vi "Maintenance v0.3.vi"(8 "Error In":errorcluster) -> (0 "Error out":errorcluster)   [LabVIEW 2017]
uses:
  GV/Maintenance GV.vi
panel:
  out "ICS_BF_Low_Level_1":bool
  in  "SOL_Index_CNVR_Output _Separator _Rear":bool
  out "RS_Measurement_2_Rear":bool
  out "RS_Measurement_3_Rear":bool
  out "RS_Measurement_4_Rear":bool
  out "RS_Measure_Clamp_Rear":bool
  in  "DO1.19":bool
  in  "Continuous?":bool
  out "DI2.25":bool
  out "DI2.26":bool
  out "DI2.31":bool
  out "DI2.30":bool
  out "DI2.29":bool
  out "DI2.28":bool
  out "DI2.27":bool
  in  "Main Tab":T1(tab)
  out "SW_Door_Front":bool
  in  "DO1.31":bool
  in  "DO1.30":bool
  out "Machine_ON":bool
  out "E_stop":bool
  out "SW_Pressure":bool
  out "SW_Start":bool
  out "SW_Reset":bool
  out "SW_Stop":bool
  out "SW_Door_Rear":bool
  out "DI1.30":bool
  out "DI1.31":bool
  out "DI2.23":bool
  out "DI2.24":bool
  in  "TL_Red":bool
  in  "TL_Orange":bool
  in  "TL_Green":bool
  in  "TL_Buzzer":bool
  out "Waveform Graph":i16[](graph)
  out "Index Time (ms)":u32
  in  "Index":bool
  out "RS_Index_Rotary_CW":bool
  out "RS_Index_Rotary_CCW":bool
  out "RS_Index_Stopper _Rear":bool
  out "PES_Index_Pallet_Sensor":bool
  out "PES_Index_Output_Part Sensor":bool
  in  "SOL_Index_Rotary_CW":bool
  in  "SOL_Index_CNVR_Rotary_CCW":bool
  in  "SOL_Index_CNVR_Stopper_Front":bool
  in  "SOL_BF2_Track1":bool
  in  "SOL_BF2_Track2":bool
  in  "SOL_BF1_Track2":bool
  in  "Bowl  Feeder_ ON 2":bool
  in  "SOL_BF_BlowerON":bool
  in  "SOL_BF1_Track1":bool
  out "ICS_BF_Pump_CNVR_Full_1":bool
  out "ICS_BF_Pump_CNVR_Full_2":bool
  out "ICS_BF_Pump_CNVR_Full_3":bool
  out "ICS_BF_Pump_CNVR_Full_4":bool
  in  "Bowl  Feeder_ ON 1":bool
  out "PES_PC_Pump Presence_1":bool
  out "PES_PC_Pump Presence_2":bool
  out "PES_PC_Pump Presence_3":bool
  out "PES_PC_Pump Presence_4":bool
  out "RS_PC_Gating_Front":bool
  out "PES_Pump_Interference":bool
  in  "SOL_Gating_CYL_Rear":bool
  in  "Pump_CNVR_Motor _ON":bool
  out "PES_TF_Low_Level":bool
  out "PES_Tube Presence_1":bool
  out "PES_Tube Presence_2":bool
  out "PES_Tube Presence_3":bool
  out "PES_Tube Presence_4":bool
  out "RS_TF_Gating CYL_Rear":bool
  out "RS_Agitatator_2_Rear":bool
  out "RS_Agitatator_1_Rear":bool
  in  "SOL_Tube_Feed_Agitator":bool
  in  "SOL_Tube_Feed_Gating_CYL":bool
  out "RS_Insertion_1_Rear":bool
  out "RS_Insertion_1_Front":bool
  out "RS_Insertion _2_Rear":bool
  out "RS_Insertion _2_Front":bool
  out "RS_Insertion _3_Rear":bool
  out "RS_Insertion _3_Front":bool
  out "RS_Insertion _4_Rear":bool
  out "RS_Insertion _4_Front":bool
  out "RS_Insertion_Clamp_Rear":bool
  in  "SOL_Insertion _CYL":bool
  in  "SOL_Insertion_Clamp_CYL":bool
  out "RS_Cutting_DNClamp _Rear":bool
  out "RS_Cutting_UPClamp _Rear":bool
  out "RS_Cutting_Rear":bool
  in  "SOL_Cutting_CYL":bool
  in  "SOL_Cutting_Clamp_CYL":bool
  in  "SOL_Insertion_Air_Nozzle":bool
  out "Distance Chart":T2(graph)
  out "IAS_MS_TubeLength_4":dbl caption="Sensor 4 (mm)" format="%#.3f"
  out "IAS_MS_TubeLength_3":dbl caption="Sensor 3 (mm)" format="%#.3f"
  out "IAS_MS_TubeLength_2":dbl caption="Sensor 2 (mm)" format="%#.3f"
  out "IAS_MS_TubeLength_1":dbl caption="Sensor 1 (mm)" format="%#.3f"
  out "RS_Measurement_1_Rear":bool
  in  "SOL_Measurement_CYL":bool
  out "RS_Rejection_1_Rear":bool
  out "RS_Rejection_2_Rear":bool
  out "RS_Rejection_3_Rear":bool
  out "RS_Rejection_4_Rear":bool
  in  "SOL_Rejection CYL_4":bool
  in  "SOL_Rejection CYL_3":bool
  in  "SOL_Rejection CYL_2":bool
  in  "SOL_Rejection CYL_1":bool
  in  "Close":bool
  # "Switches & Checks"
  # "Towerlight"
  # "Towerlight"
  # "Spare IO"
  # "Spare IO"
  # "Switches & Checks"
  # "Towerlight"
  # "Spare IO"
  # "Rotary Cylinder"
  # "Indexing"
  # "Stopper Cylinder"
  # "NOTE: This will perform a pre-defined indexing sequence while considering all safety inputs. In case of any error, no message will be shown on this screen; you will need to troubleshoot on Manual Mode."
  # "Other Inputs"
  # "Bowl Feeders"
  # "Bowl Feeder Track Full"
  # "Bowl Feeder Solenoids"
  # "Pump Conveyor Motor"
  # "Pump Presence Sensors"
  # "Gating Cylinder"
  # "Other IO"
  # "Agitator Cylinder"
  # "Tube Presence Sensors"
  # "Gating Cylinder"
  # "Other IO"
  # "Insertion Cylinders"
  # "Clamping Cylinder"
  # "Cutting Cylinder"
  # "Clamping Cylinder"
  # "Air Nozzle"
  # "Switches & Checks"
  # "Distance Measurement"
  # "Rejection Cylinder 1"
  # "Rejection Cylinder 2"
  # "Rejection Cylinder 3"
  # "Rejection Cylinder 4"
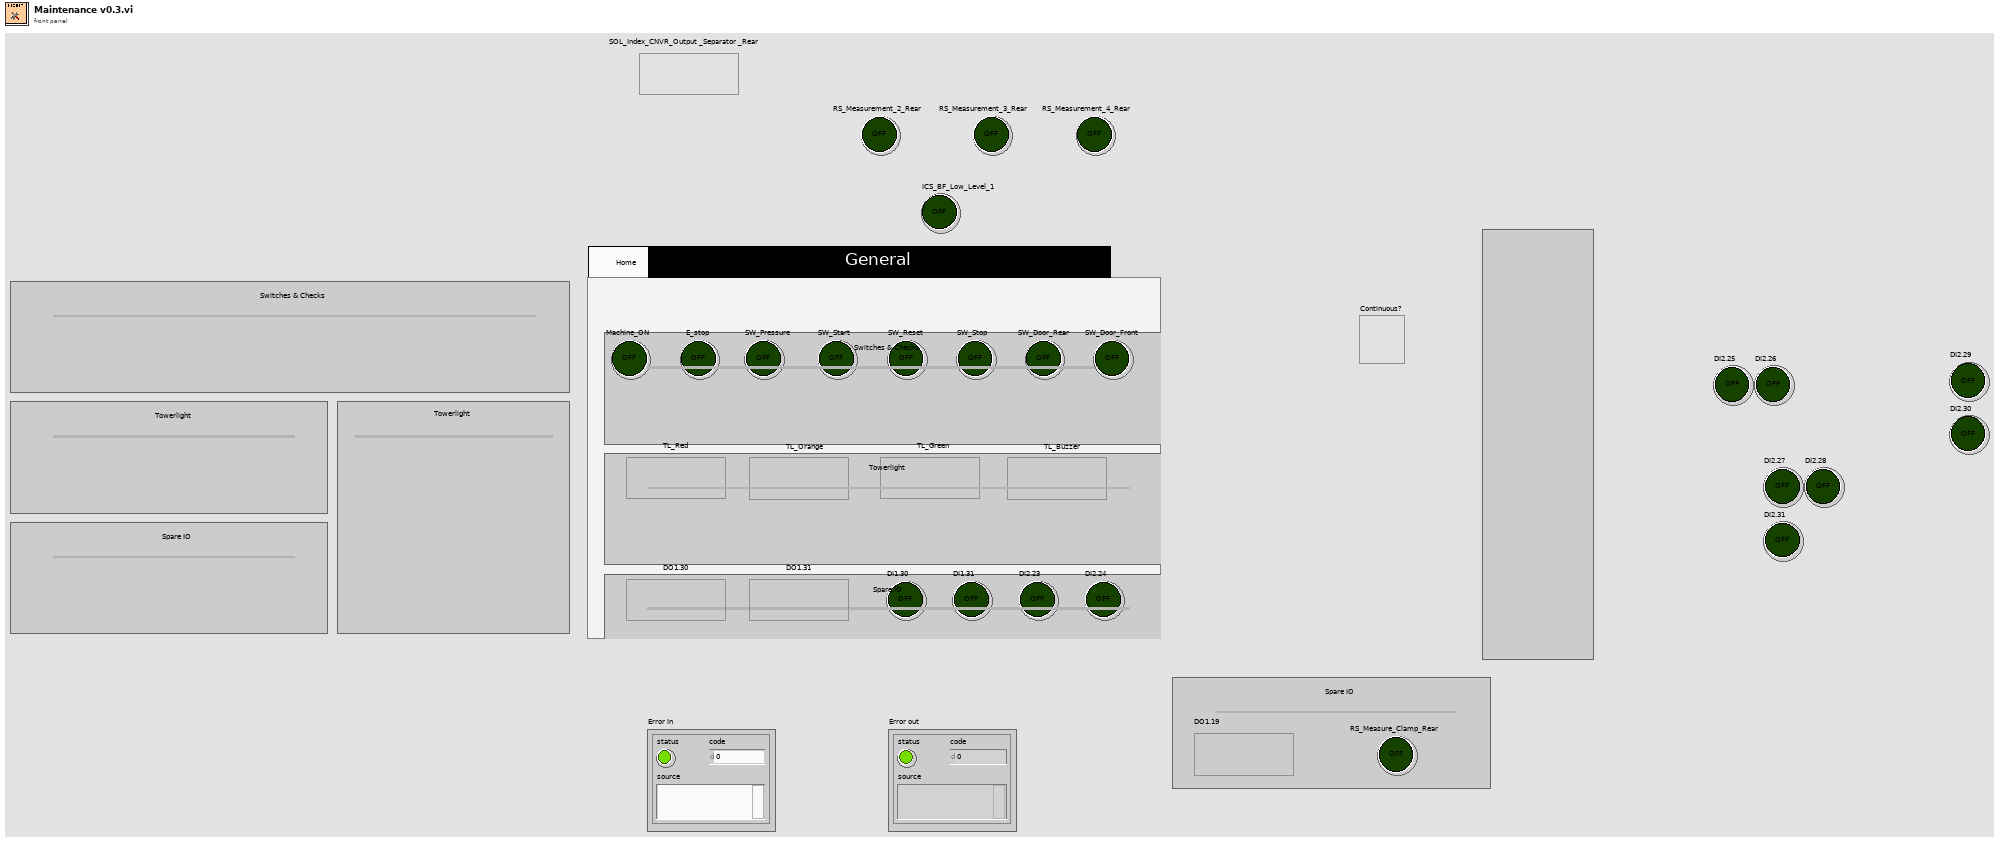
[diagram p1: front panel]
types:
  T1 = enum32{"General", "Indexing", "Bowl Feeders", "Pump Conveyor", "Tube Feeder", "Insertion Station", "Cutting Station", "Measurement Station", "Rejection Station"}
  T2 = cluster{"IAS 1":dbl, "IAS 2":dbl, "IAS 3":dbl, "IAS 4":dbl}
  T3 = typedef "All Inputs.ctl" = cluster{"DI 1":cluster{"Machine_ON":bool, "E_stop ":bool, "SW_Pressure":bool, "SW_Start ":bool, "SW_Reset":bool, "SW_Stop":bool, "SW_Door":bool, "RS_Index_Rotary_CW":bool, "RS_Index_Rotary_CCW":bool, "RS_Index_Stopper _Rear":bool, "RS_Cutting_DNClamp _Rear":bool, "PES_Index_Pallet_Sensor":bool, "PES_Index_Output_Part Sensor":bool, "ICS_BF_Low_Level_1":bool, "ICS_BF_Low_Level_2":bool, "ICS_BF_Pump_CNVR_Full_1":bool, "ICS_BF_Pump_CNVR_Full_2":bool, "ICS_BF_Pump_CNVR_Full_3":bool, "ICS_BF_Pump_CNVR_Full_4":bool, "PES_PC_Pump Presence_1":bool, "PES_PC_Pump Presence_2":bool, "PES_PC_Pump Presence_3":bool, "PES_PC_Pump Presence_4":bool, "RS_PC_Gating_Front":bool, "PES_Pump_Interference":bool, "PES_TF_Low_Level":bool, "PES_Tube Presence_1":bool, "PES_Tube Presence_2":bool, "PES_Tube Presence_3":bool, "PES_Tube Presence_4":bool, "DI1.30":bool, "DI1.31":bool}, "DI 2":cluster{"RS_Agitatator_1_Rear ":bool, "RS_Agitatator_2_Rear ":bool, "RS_TF_Gating CYL_Rear":bool, "RS_Insertion_1_Rear":bool, "RS_Insertion_1_Front":bool, "RS_Insertion _2_Rear":bool, "RS_Insertion _2_Front":bool, "RS_Insertion _3_Rear":bool, "RS_Insertion _3_Front":bool, "RS_Insertion _4_Rear":bool, "RS_Insertion _4_Front":bool, "RS_Insertion_Clamp_Rear":bool, "RS_Cutting_Rear":bool, "RS_Cutting_UPClamp _Rear":bool, "RS_Measurement_1_Rear":bool, "RS_Measurement_2_Rear":bool, "RS_Measurement_3_Rear":bool, "RS_Measurement_4_Rear":bool, "RS_Measure_Clamp_Rear":bool, "RS_Rejection_1_Rear":bool, "RS_Rejection_2_Rear":bool, "RS_Rejection_3_Rear":bool, "RS_Rejection_4_Rear":bool, "DI2.23":bool, "DI2.24":bool, "DI2.25":bool, "DI2.26":bool, "DI2.27":bool, "DI2.28":bool, "DI2.29":bool, "DI2.30":bool, "DI2.31":bool}, "IAS 1":dbl, "IAS 2":dbl, "IAS 3":dbl, "IAS 4":dbl, "DO 1":cluster{"TL_Red":bool, "TL_Orange":bool, "TL_Green":bool, "TL_Buzzer":bool, "SOL_Index_Rotary_CW":bool, "SOL_Index_CNVR_Rotary_CCW":bool, "SOL_Index_CNVR_Stopper_Rear":bool, "SOL_Index_CNVR_Output _Separator _Rear":bool, "Bowl  Feeder_ ON 1":bool, "Pump_CNVR_Motor _ON":bool, "SOL_PC_Gating_CYL_Rear":bool, "SOL_Tube_Feed_Agitatator":bool, "SOL_Tube_Feed_Gating_CYL":bool, "SOL_Insertion _CYL":bool, "SOL_Insertion_Clamp_CYL":bool, "SOL_Cutting_CYL":bool, "SOL_Cutting_Clamp_CYL":bool, "SOL_Insertion_Air_Nozzle":bool, "SOL_Measurement_CYL":bool, "DO1.19":bool, "SOL_Rejection CYL_1":bool, "SOL_Rejection CYL_2":bool, "SOL_Rejection CYL_3":bool, "SOL_Rejection CYL_4":bool, "Bowl  Feeder_ ON 2":bool, "SOL_BF_BlowerON":bool, "SOL_BF1_Track1":bool, "SOL_BF1_Track2":bool, "SOL_BF2_Track1":bool, "SOL_BF2_Track2":bool, "DO1.30":bool, "DO1.31":bool}}
  T4 = cluster{"TL_Red":bool, "TL_Orange":bool, "TL_Green":bool, "TL_Buzzer":bool, "SOL_Index_Rotary_CW":bool, "SOL_Index_CNVR_Rotary_CCW":bool, "SOL_Index_CNVR_Stopper_Rear":bool, "SOL_Index_CNVR_Output _Separator _Rear":bool, "Bowl  Feeder_ ON 1":bool, "Pump_CNVR_Motor _ON":bool, "SOL_PC_Gating_CYL_Rear":bool, "SOL_Tube_Feed_Agitatator":bool, "SOL_Tube_Feed_Gating_CYL":bool, "SOL_Insertion _CYL":bool, "SOL_Insertion_Clamp_CYL":bool, "SOL_Cutting_CYL":bool, "SOL_Cutting_Clamp_CYL":bool, "SOL_Insertion_Air_Nozzle":bool, "SOL_Measurement_CYL":bool, "DO1.19":bool, "SOL_Rejection CYL_1":bool, "SOL_Rejection CYL_2":bool, "SOL_Rejection CYL_3":bool, "SOL_Rejection CYL_4":bool, "Bowl  Feeder_ ON 2":bool, "SOL_BF_BlowerON":bool, "SOL_BF1_Track1":bool, "SOL_BF1_Track2":bool, "SOL_BF2_Track1":bool, "SOL_BF2_Track2":bool, "DO1.30":bool, "DO1.31":bool}
  T5 = typedef "Index Details.ctl" = cluster{"Time (ms)":u32, "Waveform Graph":i16[]}
  T6 = cluster{"TL_Red":bool, "TL_Orange":bool, "TL_Green":bool, "TL_Buzzer":bool, "SOL_Index_Rotary_CW":bool, "SOL_Index_CNVR_Rotary_CCW":bool, "SOL_Index_CNVR_Stopper_Rear":bool, "SOL_Index_CNVR_Output _Separator _Rear":bool, "Bowl  Feeder_ ON":bool, "Pump_CNVR_Motor _ON":bool, "SOL_Gating_CYL_Front":bool, "SOL_Tube_Feed_Agitatator":bool, "SOL_Tube_Feed_Gating_CYL":bool, "SOL_Insertion _CYL":bool, "SOL_Insertion_Clamp_CYL":bool, "SOL_Cutting_CYL":bool, "SOL_Cutting_Clamp_CYL":bool, "SOL_Insertion_Air_Nozzle":bool, "SOL_Measurement_CYL":bool, "SOL_Measure_Clamp_CYL":bool, "SOL_Rejection CYL_1":bool, "SOL_Rejection CYL_2":bool, "SOL_Rejection CYL_3":bool, "SOL_Rejection CYL_4":bool, "DO1.24":bool, "DO1.25":bool, "DO1.26":bool, "DO1.27":bool, "DO1.28":bool, "DO1.29":bool, "DO1.30":bool, "DO1.31":bool}
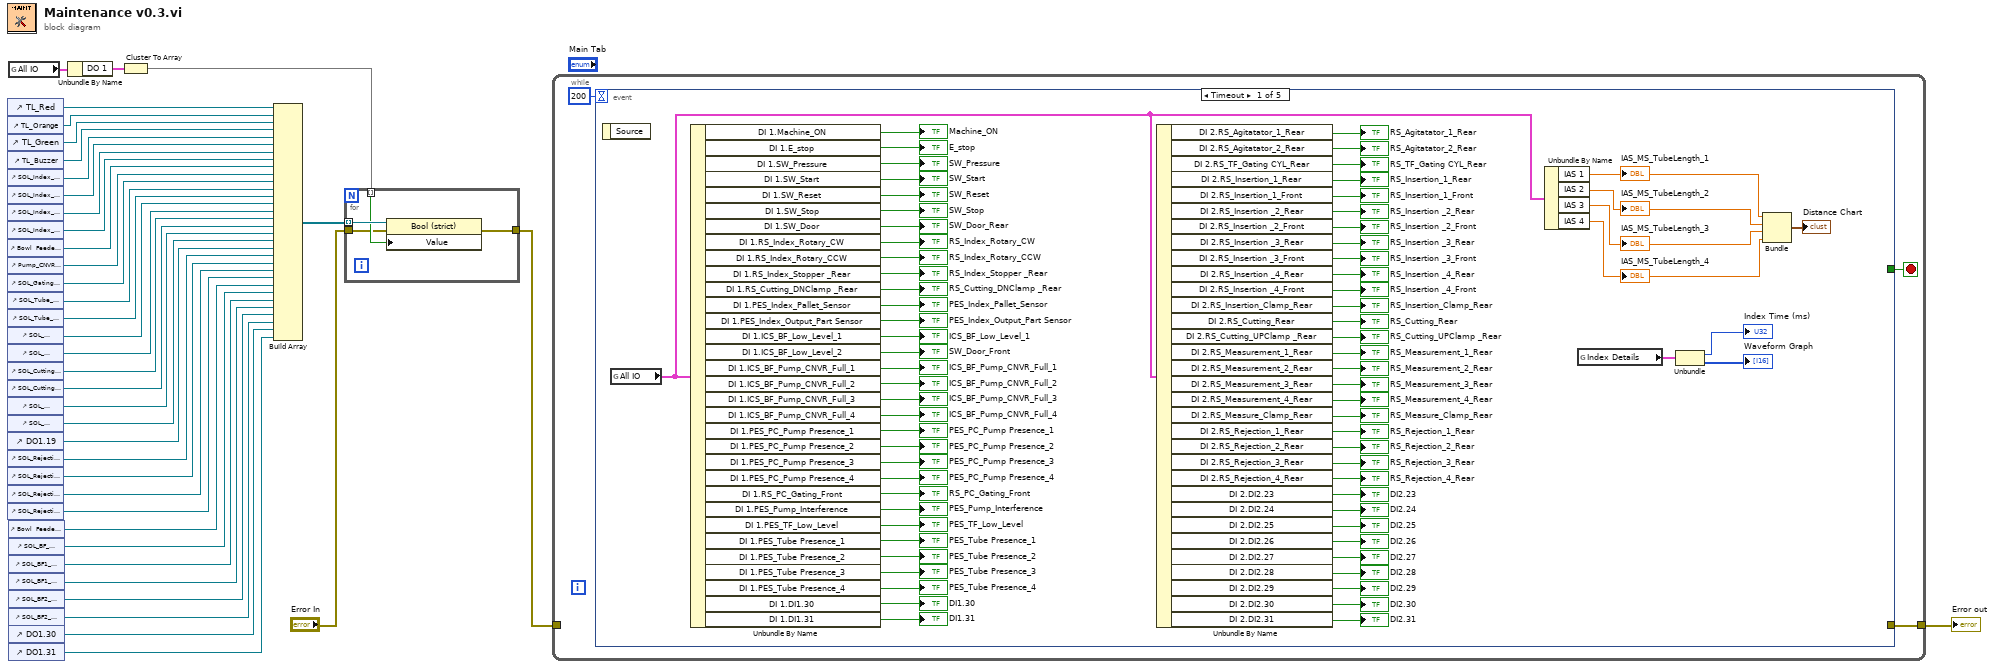
[diagram p0: block diagram]
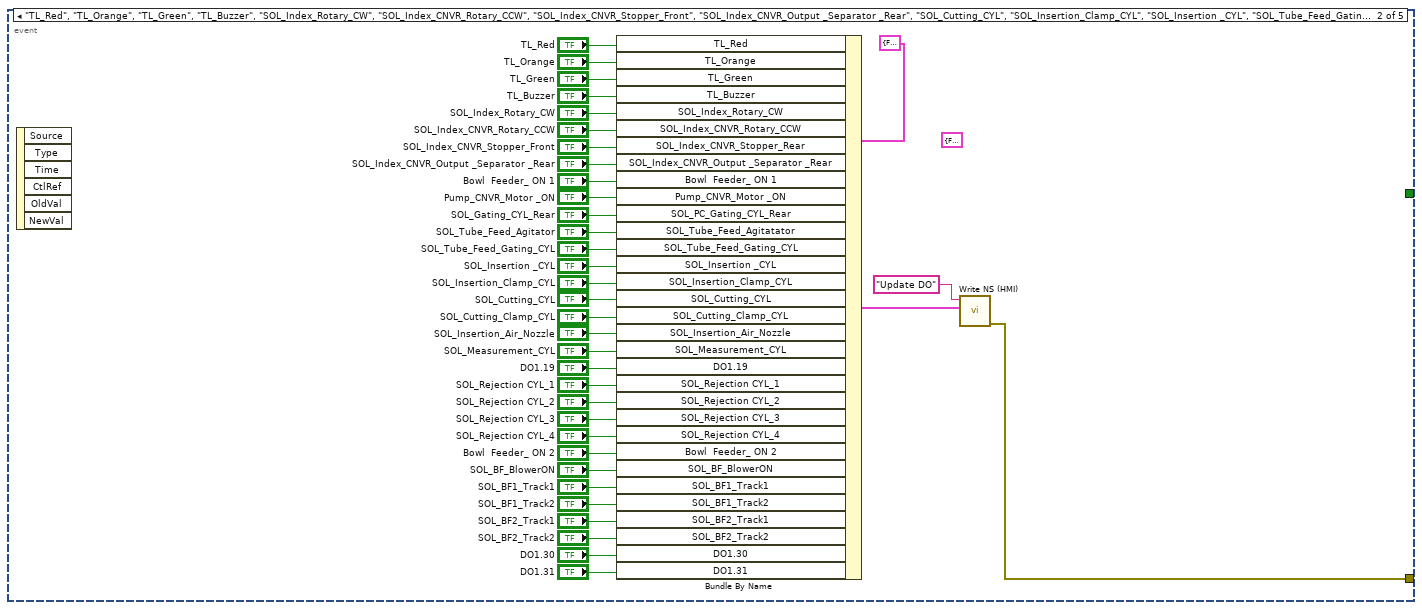
[diagram p2: hidden frame]
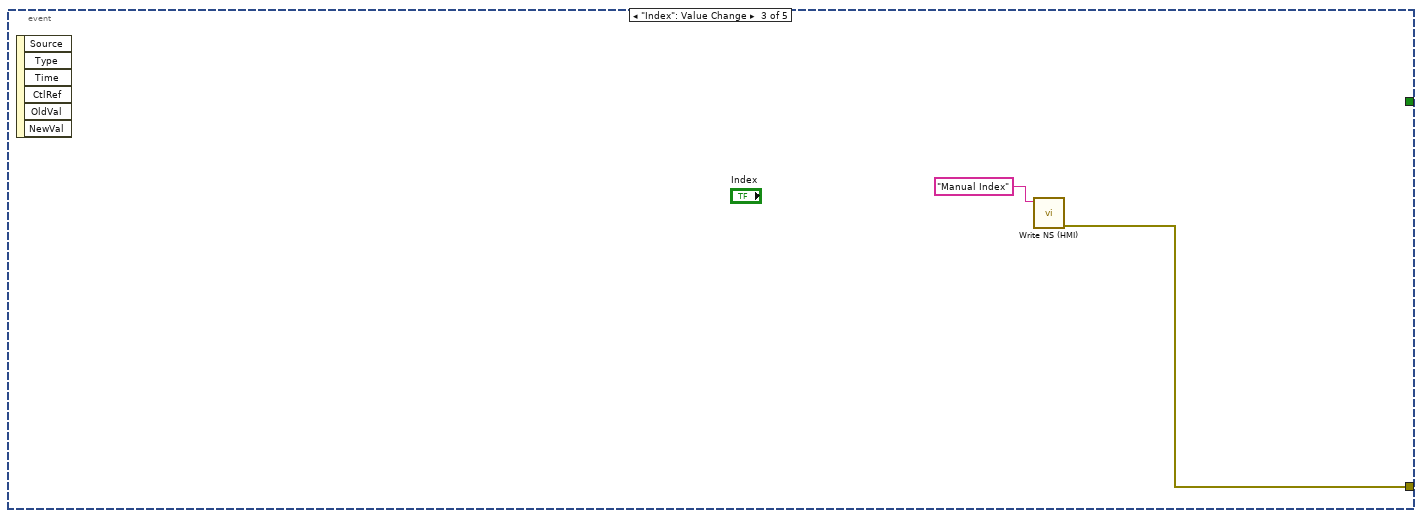
[diagram p3: hidden frame]
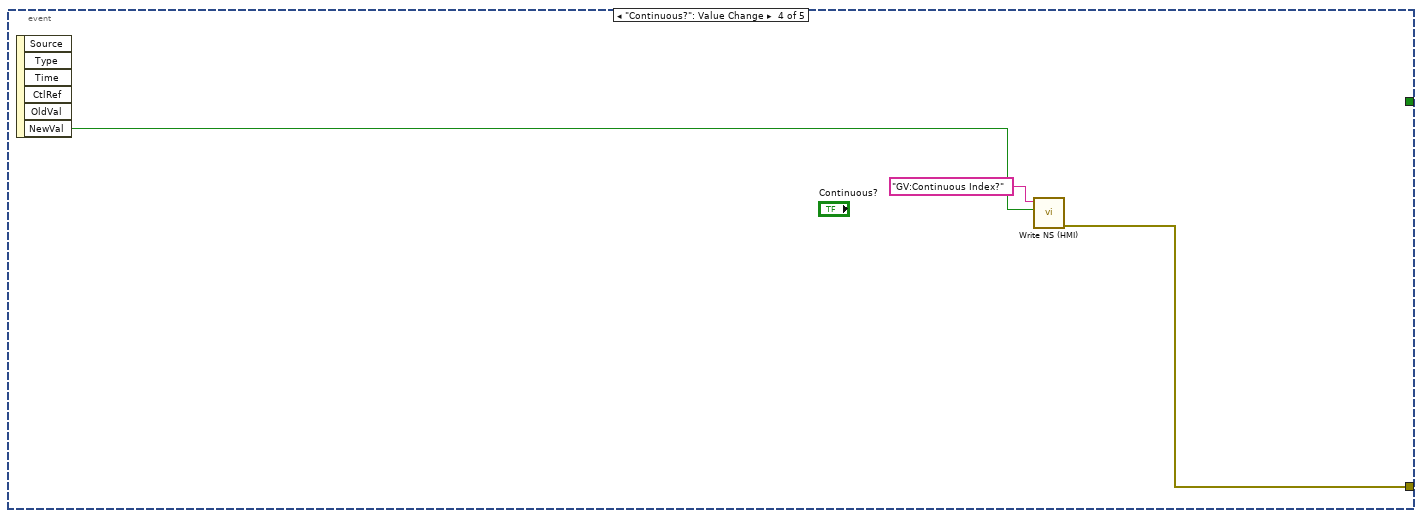
[diagram p4: hidden frame]
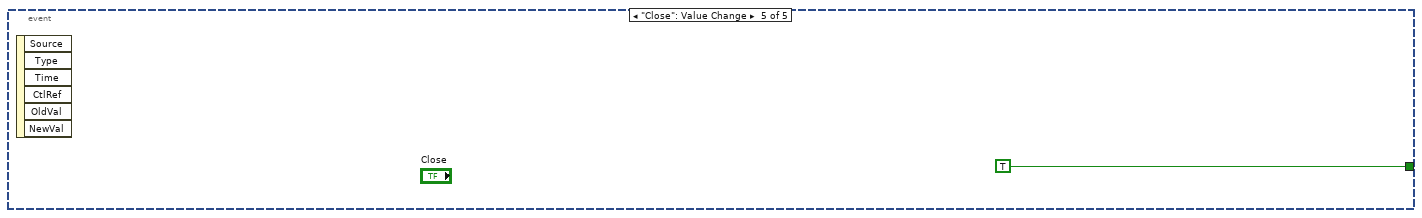
[diagram p5: hidden frame]
diagram:
  n1 = control-ref of="TL_Red"() -> (w38:refnum<vi>)
  n2 = control-ref of="TL_Orange"() -> (w37:refnum<vi>)
  n3 = control-ref of="TL_Green"() -> (w36:refnum<vi>)
  n4 = control-ref of="TL_Buzzer"() -> (w35:refnum<vi>)
  n5 = control-ref of="SOL_Index_Rotary_CW"() -> (w34:refnum<vi>)
  n6 = control-ref of="SOL_Index_CNVR_Rotary_CCW"() -> (w33:refnum<vi>)
  n7 = control-ref of="SOL_Index_CNVR_Stopper_Front"() -> (w32:refnum<vi>)
  n8 = control-ref of="SOL_Index_CNVR_Output _Separator _Rear"() -> (w31:refnum<vi>)
  n9 = control-ref of="Bowl  Feeder_ ON 1"() -> (w30:refnum<vi>)
  n10 = control-ref of="Pump_CNVR_Motor _ON"() -> (w29:refnum<vi>)
  n11 = control-ref of="SOL_Gating_CYL_Rear"() -> (w28:refnum<vi>)
  n12 = control-ref of="SOL_Tube_Feed_Agitator"() -> (w27:refnum<vi>)
  n13 = control-ref of="SOL_Tube_Feed_Gating_CYL"() -> (w26:refnum<vi>)
  n14 = control-ref of="SOL_Insertion _CYL"() -> (w25:refnum<vi>)
  n15 = control-ref of="SOL_Insertion_Clamp_CYL"() -> (w24:refnum<vi>)
  n16 = control-ref of="SOL_Cutting_CYL"() -> (w23:refnum<vi>)
  n17 = control-ref of="SOL_Cutting_Clamp_CYL"() -> (w22:refnum<vi>)
  n18 = control-ref of="SOL_Insertion_Air_Nozzle"() -> (w21:refnum<vi>)
  n19 = control-ref of="SOL_Measurement_CYL"() -> (w20:refnum<vi>)
  n20 = control-ref of="DO1.19"() -> (w19:refnum<vi>)
  n21 = control-ref of="SOL_Rejection CYL_1"() -> (w18:refnum<vi>)
  n22 = control-ref of="SOL_Rejection CYL_2"() -> (w17:refnum<vi>)
  n23 = control-ref of="SOL_Rejection CYL_3"() -> (w16:refnum<vi>)
  n24 = control-ref of="SOL_Rejection CYL_4"() -> (w15:refnum<vi>)
  n25 = global read "Maintenance GV.vi" "All IO"() -> (w5:T3)
  n26 = control-ref of="Bowl  Feeder_ ON 2"() -> (w14:refnum<vi>)
  n27 = control-ref of="SOL_BF_BlowerON"() -> (w13:refnum<vi>)
  n28 = control-ref of="SOL_BF1_Track1"() -> (w12:refnum<vi>)
  n29 = control-ref of="SOL_BF1_Track2"() -> (w11:refnum<vi>)
  n30 = control-ref of="SOL_BF2_Track1"() -> (w10:refnum<vi>)
  n31 = control-ref of="SOL_BF2_Track2"() -> (w9:refnum<vi>)
  n32 = control-ref of="DO1.30"() -> (w8:refnum<vi>)
  n33 = control-ref of="DO1.31"() -> (w7:refnum<vi>)
  n34 = Unbundle By Name(w5) -> ("DO 1"=w4:T4)
  n35 = Cluster To Array(cluster=w4) -> (array=w3:bool[])
  n36 = Build Array(w38, w37, w36, w35, w34, w33, w32, w31, w30, w29, w28, w27, w26, w25, w24, w23, w22, w21, w20, w19, w18, w17, w16, w15, w14, w13, w12, w11, w10, w9, w8, w7) -> (w6:refnum<vi>[])
  n37 = for {
    tunnel: w6 -> [w43] mode=indexing
    tunnel: w3 -> [w42] mode=indexing
    tunnel: "Error In" -> [w41]
    tunnel: [w40] -> w1
    n38 = property class="Bool (strict)"(reference=w43, error in=w41, "Value"=w42) -> (error out=w40:errorcluster)  [unwired: 1 out]
  }
  n39 = while {
    tunnel: [w44] -> w39
    tunnel: w1 -> [_]
    stop <- w45 stop-if-true
    n40 = event shown="[0] Timeout" {
      selector: _ -> [_ _ _ _ _]
      dyn-events: _ -> [_ _ _ _ _]
      timeout: 200 -> [_ _ _ _ _]
      tunnel: [_ _ _ _ TRUE] -> w45
      tunnel: [_ w122 w156 w159 _] -> w44
      event Timeout {
        n41 = event-data() -> ()  [unwired: 1 in, 1 out]
        n42 = global read "Maintenance GV.vi" "All IO"() -> (w50:T3)
        n43 = Unbundle By Name(w50) -> ("DI 1.Machine_ON"=→"Machine_ON":bool, "DI 1.E_stop"=→"E_stop":bool, "DI 1.SW_Pressure"=→"SW_Pressure":bool, "DI 1.SW_Start"=→"SW_Start":bool, "DI 1.SW_Reset"=→"SW_Reset":bool, "DI 1.SW_Stop"=→"SW_Stop":bool, "DI 1.SW_Door"=→"SW_Door_Rear":bool, "DI 1.RS_Index_Rotary_CW"=→"RS_Index_Rotary_CW":bool, "DI 1.RS_Index_Rotary_CCW"=→"RS_Index_Rotary_CCW":bool, "DI 1.RS_Index_Stopper _Rear"=→"RS_Index_Stopper _Rear":bool, "DI 1.RS_Cutting_DNClamp _Rear"=→"RS_Cutting_DNClamp _Rear":bool, "DI 1.PES_Index_Pallet_Sensor"=→"PES_Index_Pallet_Sensor":bool, "DI 1.PES_Index_Output_Part Sensor"=→"PES_Index_Output_Part Sensor":bool, "DI 1.ICS_BF_Low_Level_1"=→"ICS_BF_Low_Level_1":bool, "DI 1.ICS_BF_Low_Level_2"=→"SW_Door_Front":bool, "DI 1.ICS_BF_Pump_CNVR_Full_1"=→"ICS_BF_Pump_CNVR_Full_1":bool, "DI 1.ICS_BF_Pump_CNVR_Full_2"=→"ICS_BF_Pump_CNVR_Full_2":bool, "DI 1.ICS_BF_Pump_CNVR_Full_3"=→"ICS_BF_Pump_CNVR_Full_3":bool, "DI 1.ICS_BF_Pump_CNVR_Full_4"=→"ICS_BF_Pump_CNVR_Full_4":bool, "DI 1.PES_PC_Pump Presence_1"=→"PES_PC_Pump Presence_1":bool, "DI 1.PES_PC_Pump Presence_2"=→"PES_PC_Pump Presence_2":bool, "DI 1.PES_PC_Pump Presence_3"=→"PES_PC_Pump Presence_3":bool, "DI 1.PES_PC_Pump Presence_4"=→"PES_PC_Pump Presence_4":bool, "DI 1.RS_PC_Gating_Front"=→"RS_PC_Gating_Front":bool, "DI 1.PES_Pump_Interference"=→"PES_Pump_Interference":bool, "DI 1.PES_TF_Low_Level"=→"PES_TF_Low_Level":bool, "DI 1.PES_Tube Presence_1"=→"PES_Tube Presence_1":bool, "DI 1.PES_Tube Presence_2"=→"PES_Tube Presence_2":bool, "DI 1.PES_Tube Presence_3"=→"PES_Tube Presence_3":bool, "DI 1.PES_Tube Presence_4"=→"PES_Tube Presence_4":bool, "DI 1.DI1.30"=→"DI1.30":bool, "DI 1.DI1.31"=→"DI1.31":bool)
        n44 = Unbundle By Name(w50) -> ("DI 2.RS_Agitatator_1_Rear"=→"RS_Agitatator_1_Rear":bool, "DI 2.RS_Agitatator_2_Rear"=→"RS_Agitatator_2_Rear":bool, "DI 2.RS_TF_Gating CYL_Rear"=→"RS_TF_Gating CYL_Rear":bool, "DI 2.RS_Insertion_1_Rear"=→"RS_Insertion_1_Rear":bool, "DI 2.RS_Insertion_1_Front"=→"RS_Insertion_1_Front":bool, "DI 2.RS_Insertion _2_Rear"=→"RS_Insertion _2_Rear":bool, "DI 2.RS_Insertion _2_Front"=→"RS_Insertion _2_Front":bool, "DI 2.RS_Insertion _3_Rear"=→"RS_Insertion _3_Rear":bool, "DI 2.RS_Insertion _3_Front"=→"RS_Insertion _3_Front":bool, "DI 2.RS_Insertion _4_Rear"=→"RS_Insertion _4_Rear":bool, "DI 2.RS_Insertion _4_Front"=→"RS_Insertion _4_Front":bool, "DI 2.RS_Insertion_Clamp_Rear"=→"RS_Insertion_Clamp_Rear":bool, "DI 2.RS_Cutting_Rear"=→"RS_Cutting_Rear":bool, "DI 2.RS_Cutting_UPClamp _Rear"=→"RS_Cutting_UPClamp _Rear":bool, "DI 2.RS_Measurement_1_Rear"=→"RS_Measurement_1_Rear":bool, "DI 2.RS_Measurement_2_Rear"=→"RS_Measurement_2_Rear":bool, "DI 2.RS_Measurement_3_Rear"=→"RS_Measurement_3_Rear":bool, "DI 2.RS_Measurement_4_Rear"=→"RS_Measurement_4_Rear":bool, "DI 2.RS_Measure_Clamp_Rear"=→"RS_Measure_Clamp_Rear":bool, "DI 2.RS_Rejection_1_Rear"=→"RS_Rejection_1_Rear":bool, "DI 2.RS_Rejection_2_Rear"=→"RS_Rejection_2_Rear":bool, "DI 2.RS_Rejection_3_Rear"=→"RS_Rejection_3_Rear":bool, "DI 2.RS_Rejection_4_Rear"=→"RS_Rejection_4_Rear":bool, "DI 2.DI2.23"=→"DI2.23":bool, "DI 2.DI2.24"=→"DI2.24":bool, "DI 2.DI2.25"=→"DI2.25":bool, "DI 2.DI2.26"=→"DI2.26":bool, "DI 2.DI2.27"=→"DI2.27":bool, "DI 2.DI2.28"=→"DI2.28":bool, "DI 2.DI2.29"=→"DI2.29":bool, "DI 2.DI2.30"=→"DI2.30":bool, "DI 2.DI2.31"=→"DI2.31":bool)
        n45 = Unbundle By Name(w50) -> ("IAS 1"=w110:dbl, "IAS 2"=w109:dbl, "IAS 3"=w108:dbl, "IAS 4"=w107:dbl)
        "IAS_MS_TubeLength_1" <- w110
        "IAS_MS_TubeLength_2" <- w109
        "IAS_MS_TubeLength_3" <- w108
        "IAS_MS_TubeLength_4" <- w107
        n46 = global read "Maintenance GV.vi" "Index Details"() -> (w49:T5)
        n47 = Unbundle(w49) -> ("Time (ms)"=→"Index Time (ms)":u32, "Waveform Graph"=→"Waveform Graph":i16[])
        n48 = Bundle("IAS 1"=w110, "IAS 2"=w109, "IAS 3"=w108, "IAS 4"=w107) -> (→"Distance Chart":T2)  [unwired: 1 in]
      }
      event "TL_Red", "TL_Orange", "TL_Green", "TL_Buzzer", "SOL_Index_Rotary_CW", "SOL_Index_CNVR_Rotary_CCW", "SOL_Index_CNVR_Stopper_Front", "SOL_Index_CNVR_Output _Separator _Rear", "SOL_Cutting_CYL", "SOL_Insertion_Clamp_CYL", "SOL_Insertion _CYL", "SOL_Tube_Feed_Gating_CYL", "SOL_Tube_Feed_Agitator", "SOL_Gating_CYL_Rear", "Pump_CNVR_Motor _ON", "Bowl  Feeder_ ON 1", "SOL_Rejection CYL_4", "SOL_Rejection CYL_3", "SOL_Rejection CYL_2", "SOL_Rejection CYL_1", "DO1.19", "SOL_Measurement_CYL", "SOL_Insertion_Air_Nozzle", "SOL_Cutting_Clamp_CYL", "DO1.31", "DO1.30", "SOL_BF2_Track2", "SOL_BF2_Track1", "SOL_BF1_Track2", "SOL_BF1_Track1", "SOL_BF_BlowerON", "Bowl  Feeder_ ON 2": Value Change {
        (unwired) T6 {"TL_Red"=FALSE, "TL_Orange"=FALSE, "TL_Green"=FALSE, "TL_Buzzer"=FALSE, "SOL_Index_Rotary_CW"=FALSE, "SOL_Index_CNVR_Rotary_CCW"=FALSE, "SOL_Index_CNVR_Stopper_Rear"=FALSE, "SOL_Index_CNVR_Output _Separator _Rear"=FALSE, "Bowl  Feeder_ ON"=FALSE, "Pump_CNVR_Motor _ON"=FALSE, "SOL_Gating_CYL_Front"=FALSE, "SOL_Tube_Feed_Agitatator"=FALSE, "SOL_Tube_Feed_Gating_CYL"=FALSE, "SOL_Insertion _CYL"=FALSE, "SOL_Insertion_Clamp_CYL"=FALSE, "SOL_Cutting_CYL"=FALSE, "SOL_Cutting_Clamp_CYL"=FALSE, "SOL_Insertion_Air_Nozzle"=FALSE, "SOL_Measurement_CYL"=FALSE, "SOL_Measure_Clamp_CYL"=FALSE, "SOL_Rejection CYL_1"=FALSE, "SOL_Rejection CYL_2"=FALSE, "SOL_Rejection CYL_3"=FALSE, "SOL_Rejection CYL_4"=FALSE, "DO1.24"=FALSE, "DO1.25"=FALSE, "DO1.26"=FALSE, "DO1.27"=FALSE, "DO1.28"=FALSE, "DO1.29"=FALSE, "DO1.30"=FALSE, "DO1.31"=FALSE} ("DO 1")
        n49 = event-data() -> ()  [unwired: 1 in, 6 out]
        n50 = Bundle By Name(cluster=T4 {"TL_Red"=FALSE, "TL_Orange"=FALSE, "TL_Green"=FALSE, "TL_Buzzer"=FALSE, "SOL_Index_Rotary_CW"=FALSE, "SOL_Index_CNVR_Rotary_CCW"=FALSE, "SOL_Index_CNVR_Stopper_Rear"=FALSE, "SOL_Index_CNVR_Output _Separator _Rear"=FALSE, "Bowl  Feeder_ ON 1"=FALSE, "Pump_CNVR_Motor _ON"=FALSE, "SOL_PC_Gating_CYL_Rear"=FALSE, "SOL_Tube_Feed_Agitatator"=FALSE, "SOL_Tube_Feed_Gating_CYL"=FALSE, "SOL_Insertion _CYL"=FALSE, "SOL_Insertion_Clamp_CYL"=FALSE, "SOL_Cutting_CYL"=FALSE, "SOL_Cutting_Clamp_CYL"=FALSE, "SOL_Insertion_Air_Nozzle"=FALSE, "SOL_Measurement_CYL"=FALSE, "DO1.19"=FALSE, "SOL_Rejection CYL_1"=FALSE, "SOL_Rejection CYL_2"=FALSE, "SOL_Rejection CYL_3"=FALSE, "SOL_Rejection CYL_4"=FALSE, "Bowl  Feeder_ ON 2"=FALSE, "SOL_BF_BlowerON"=FALSE, "SOL_BF1_Track1"=FALSE, "SOL_BF1_Track2"=FALSE, "SOL_BF2_Track1"=FALSE, "SOL_BF2_Track2"=FALSE, "DO1.30"=FALSE, "DO1.31"=FALSE} ("DO 1"), "TL_Red"="TL_Red", "TL_Orange"="TL_Orange", "TL_Green"="TL_Green", "TL_Buzzer"="TL_Buzzer", "SOL_Index_Rotary_CW"="SOL_Index_Rotary_CW", "SOL_Index_CNVR_Rotary_CCW"="SOL_Index_CNVR_Rotary_CCW", "SOL_Index_CNVR_Stopper_Rear"="SOL_Index_CNVR_Stopper_Front", "SOL_Index_CNVR_Output _Separator _Rear"="SOL_Index_CNVR_Output _Separator _Rear", "Bowl  Feeder_ ON 1"="Bowl  Feeder_ ON 1", "Pump_CNVR_Motor _ON"="Pump_CNVR_Motor _ON", "SOL_PC_Gating_CYL_Rear"="SOL_Gating_CYL_Rear", "SOL_Tube_Feed_Agitatator"="SOL_Tube_Feed_Agitator", "SOL_Tube_Feed_Gating_CYL"="SOL_Tube_Feed_Gating_CYL", "SOL_Insertion _CYL"="SOL_Insertion _CYL", "SOL_Insertion_Clamp_CYL"="SOL_Insertion_Clamp_CYL", "SOL_Cutting_CYL"="SOL_Cutting_CYL", "SOL_Cutting_Clamp_CYL"="SOL_Cutting_Clamp_CYL", "SOL_Insertion_Air_Nozzle"="SOL_Insertion_Air_Nozzle", "SOL_Measurement_CYL"="SOL_Measurement_CYL", "DO1.19"="DO1.19", "SOL_Rejection CYL_1"="SOL_Rejection CYL_1", "SOL_Rejection CYL_2"="SOL_Rejection CYL_2", "SOL_Rejection CYL_3"="SOL_Rejection CYL_3", "SOL_Rejection CYL_4"="SOL_Rejection CYL_4", "Bowl  Feeder_ ON 2"="Bowl  Feeder_ ON 2", "SOL_BF_BlowerON"="SOL_BF_BlowerON", "SOL_BF1_Track1"="SOL_BF1_Track1", "SOL_BF1_Track2"="SOL_BF1_Track2", "SOL_BF2_Track1"="SOL_BF2_Track1", "SOL_BF2_Track2"="SOL_BF2_Track2", "DO1.30"="DO1.30", "DO1.31"="DO1.31") -> (w133:T4)
        n51 = call "Write NS (HMI).vi"("Message Data"=w133, "Message"="Update DO") -> ("error out"=w122:errorcluster)  [unwired: 9 in]
      }
      event "Index": Value Change {
        n52 = event-data() -> ()  [unwired: 1 in, 6 out]
        n53 = call "Write NS (HMI).vi"("Message"="Manual Index") -> ("error out"=w156:errorcluster)  [unwired: 10 in]
      }
      event "Continuous?": Value Change {
        n54 = event-data() -> ("NewVal"=w158:bool)  [unwired: 1 in, 5 out]
        n55 = call "Write NS (HMI).vi"("Message Data"=w158, "Message"="GV:Continuous Index?") -> ("error out"=w159:errorcluster)  [unwired: 9 in]
      }
      event "Close": Value Change {
        n56 = event-data() -> ()  [unwired: 1 in, 6 out]
      }
    }
  }
  "Error out" <- w39
